vi "Set Page Displayed.vi"(8 "error in (no error)":errorcluster, 11 "Page to display":T1) -> (0 "error out":errorcluster)   [LabVIEW 2019]
uses:
  Comms/State Controller/Controls/Comms Loop States.ctl
  Controls/Pages Tab.ctl
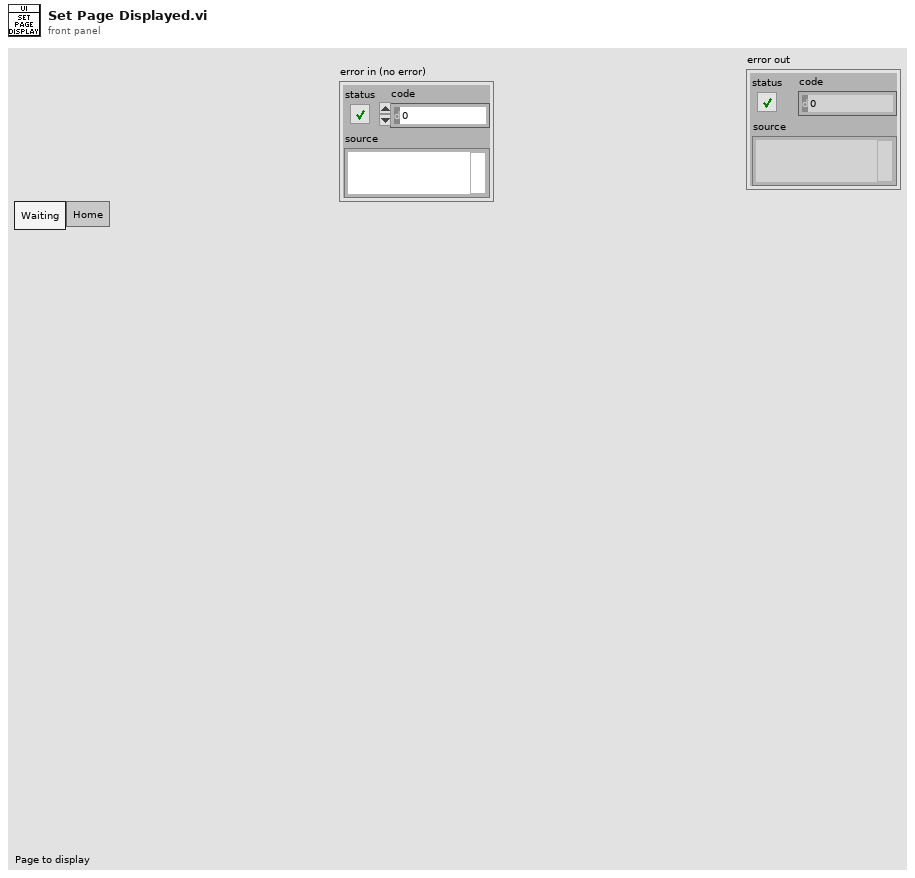
[diagram p1: front panel]
types:
  T1 = typedef "Pages Tab.ctl" = enum32{"Waiting", "Home"}
  T2 = typedef "Comms Loop States.ctl" = enum16{"Initalise", "User Event", "HEART_BEAT", "SEND_LOG_FILE_NAME", "Clear Log File Names", "SEND_LOG_FILE_CHUNK", "SEND_LOG_FILE_SIZE", "SEND_SD_CARD_INFO", "SEND_BATTERY_INFO", "SEND_LOGGING_PERIOD", "SEND_RTC_TIME", "SEND_CURRENT_MEASUREMENTS", "ERROR_MSG", "Clear Error Messages", "Send Message", "Idle", "Sensor Connected", "Sensor Disconnected", "Set Page Displayed"}
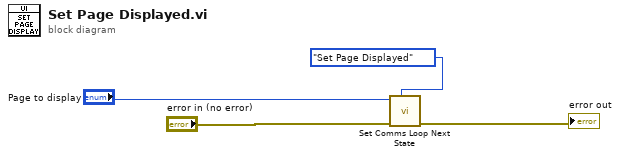
[diagram p0: block diagram]
diagram:
  n1 = call "Set Comms Loop Next State.vi"("Command"=Comms_Loop_States."Set Page Displayed", "error in (no error)"="error in (no error)", "Data"="Page to display") -> ("error out"=→"error out":errorcluster)  [unwired: 8 in]
